vi "Set Document Source.vi"(8 "Error In":errorcluster, 10 "Document Source":string, 11 "WebView in":refnum<class "WebView.lvclass">) -> (0 "Error Out":errorcluster, 3 "WebView out":refnum<class "WebView.lvclass">)   [LabVIEW 2020, in "WebView.lvclass"]
uses:
  WebView.lvclass
  WebView.lvclass/WebView.ctl
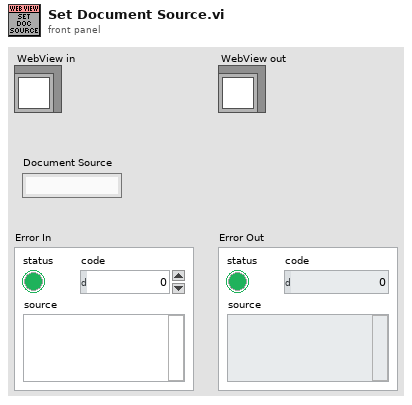
[diagram p1: front panel]
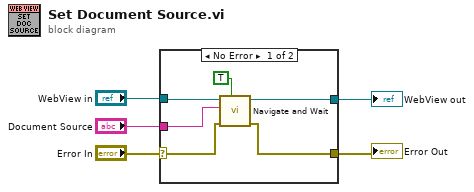
[diagram p0: block diagram]
diagram:
  n1 = case shown="No Error" "Error In" {
    selector: "Error In" -> [w8 w13]
    tunnel: [w7 w13] -> w4
    tunnel: [w10 w12] -> w2
    tunnel: "WebView in" -> [w9 w12]
    tunnel: "Document Source" -> [w11 _]
    frame No Error {
      n2 = call "Navigate and Wait.vi"("html Source (URL)"=TRUE, "Error In"=w8, "Source"=w11, "WebView in"=w9) -> ("Error Out"=w7:errorcluster, "WebView out"=w10:refnum<class "WebView.lvclass">)  [unwired: 5 in, 1 out]
    }
    frame Error {
    }
  }
  "Error Out" <- w4
  "WebView out" <- w2
